vi "DataForPython.vi"() -> ()   [LabVIEW 2016]
panel:
  out "Texto":string
  in  "PrimeiroCanal":i32=1
  in  "MaxFreq":dbl=200.0
  in  "TestDir":path=path "L:/Documentos/Programas em LabVIEW/Programas funcionais/GradesSaltoCaxias/Data/01_ENSAIO" caption="Pasta do ensaio"
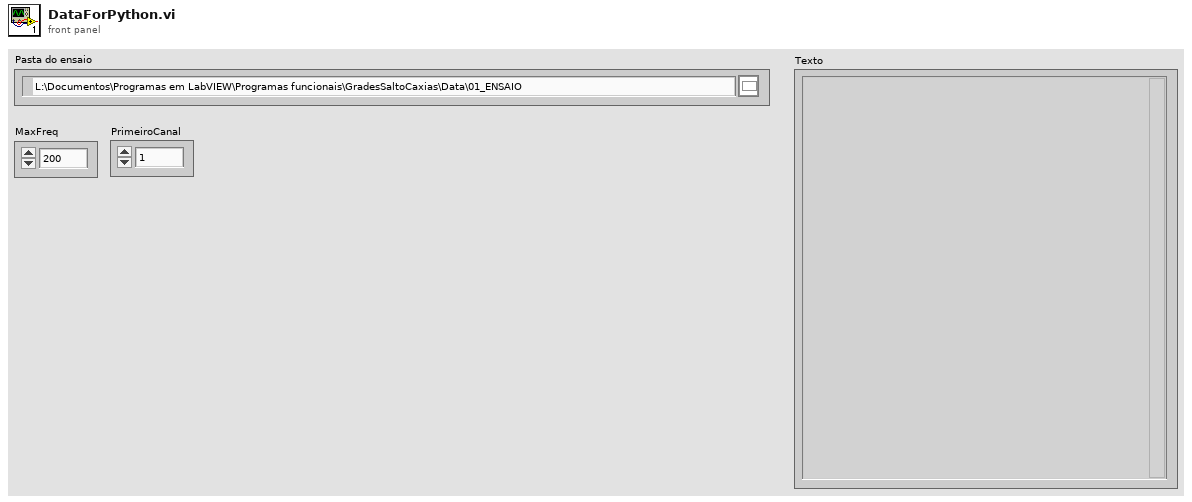
[diagram p1: front panel]
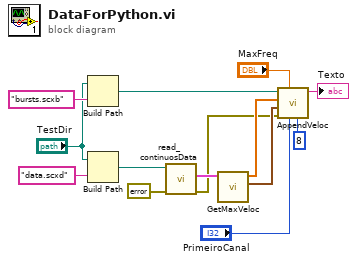
[diagram p0: block diagram]
diagram:
  n1 = Build Path(base path="TestDir", name or relative path="bursts.scxb") -> (appended path=w9:path)
  n2 = Build Path(base path="TestDir", name or relative path="data.scxd") -> (appended path=w13:path)
  n3 = call "read_continuosData.vi"("error in"=errorcluster {"status"=FALSE, "code"=0, "source"=""}, "DirPath"=w13) -> ("error out"=w5:errorcluster, "CurrenMeters"=w10:cluster{"Array":timestamp[], "Array":dbl[]}[])  [unwired: 7 in, 1 out]
  n4 = call "GetMaxVeloc.vi"("CurrenMeters"=w10) -> ("TimeStamps"=w6:timestamp[], "MaxVelocs"=w7:dbl[])  [unwired: 9 in]
  n5 = call "AppendVeloc.vi"("GroupSize"=8, "PrimeiroCanal"="PrimeiroCanal", "MaxFreq"="MaxFreq", "error in"=w5, "VelocTimeStamps"=w6, "MaxVelocs"=w7, "DirPath"=w9) -> ("Texto"=→"Texto":string)  [unwired: 3 in, 1 out]
